vi "led_player.vi"() -> ()   [LabVIEW 2022 SP3]
uses:
  <vilib>/DAQmx/write.llb/DAQmx Write (Digital 1D Bool 1Chan 1Samp).vi
  <vilib>/DAQmx/create/channels.llb/DAQmx Create Channel (DO-Digital Output).vi
  <vilib>/DAQmx/create/channels.llb/DAQmx Create Channel (CO-Pulse Generation-Time).vi
  <vilib>/DAQmx/configure/trigger.llb/DAQmx Start Trigger (Digital Edge).vi
  <vilib>/DAQmx/miscellaneous.llb/DAQmx Fill In Error Info.vi
panel:
  in  "Numeric":i32
  out "Array":bool[](array[boolean])
  out "task done?":bool
  in  "counter":tag="cDAQ2/_ctr0"
  in  "source":tag="/cDAQ2/PFI0"
  in  "lines":tag="cDAQ2Mod3/port0/line0:3"
  in  "stop":bool
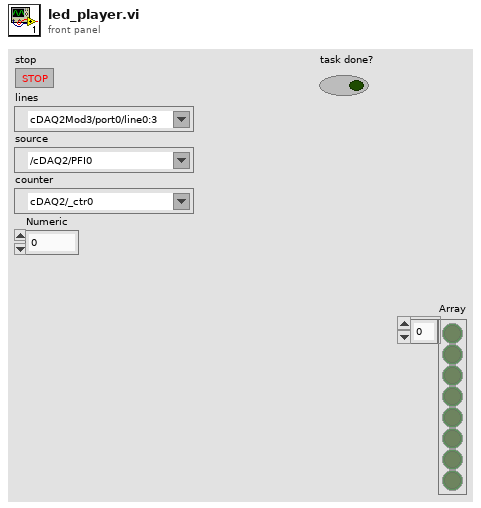
[diagram p1: front panel]
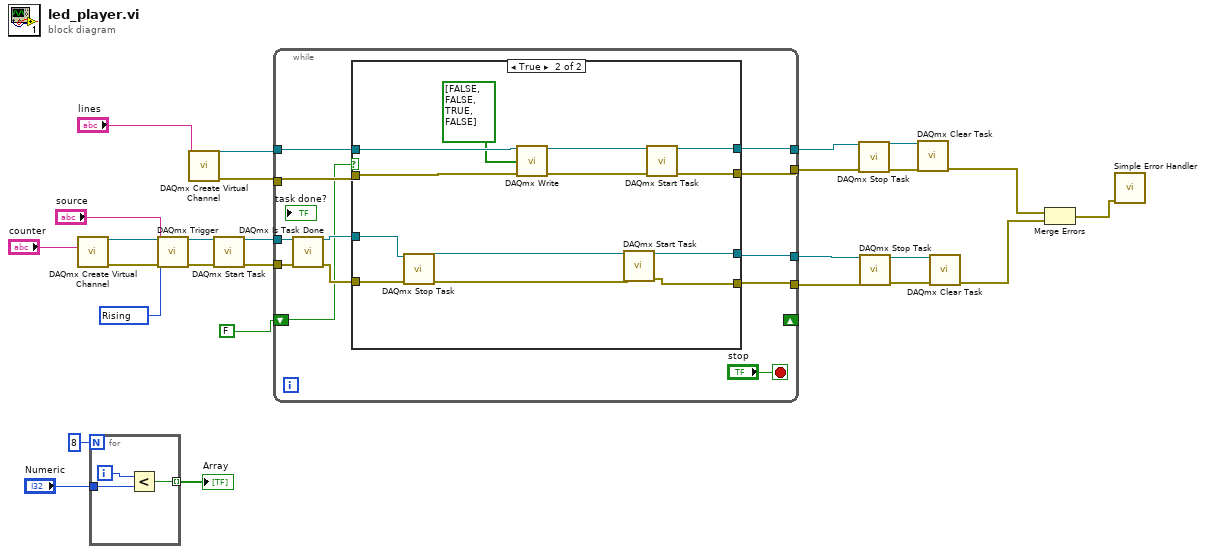
[diagram p0: block diagram]
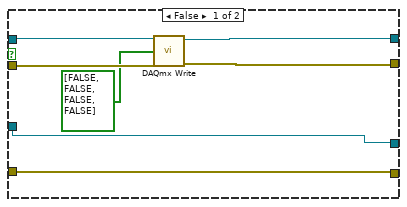
[diagram p2: hidden frame]
diagram:
  w6 = 10280 items=["Rising"=10280, "Falling"=10171] ("edge")
  n1 = call-poly <vilib>:"DAQmx Create Virtual Channel.vi"("counter"="counter") -> ("task out"=w16:refnum<k21>, "error out"=w27:errorcluster)  [unwired: 13 in]
  n2 = for {
    N: 8 -> [_]
    tunnel: "Numeric" -> [w29]
    tunnel: [w28] -> w3 mode=indexing
    i -> [w30]
    n3 = Less?(x=w30, y=w29) -> (x < y?=w28:bool)
  }
  "Array" <- w3
  n4 = call-poly <vilib>:"DAQmx Trigger.vi"("task/channels in"=w16, "source"="source", "edge"=w6, "error in"=w27) -> ("task out"=w17:refnum<k21>, "error out"=w26:errorcluster)  [unwired: 10 in]
  n5 = call-poly <vilib>:"DAQmx Create Virtual Channel.vi"("lines"="lines") -> ("task out"=w9:refnum<k21>, "error out"=w15:errorcluster)  [unwired: 13 in]
  n6 = call <vilib>:"DAQmx Start Task.vi"("task/channels in"=w17, "error in"=w26) -> ("task out"=w18:refnum<k21>, "error out"=w25:errorcluster)  [unwired: 12 in]
  n7 = while {
    tunnel: w25 -> [w42]
    tunnel: [w40] -> w24
    tunnel: [w39] -> w19
    tunnel: w18 -> [w37]
    tunnel: w15 -> [w36]
    tunnel: [w35] -> w14
    tunnel: [w34] -> w10
    tunnel: w9 -> [w33]
    shift-right: _ -> [_]
    shift-left: FALSE -> [w31]
    stop <- "stop" stop-if-true
    n8 = call <vilib>:"DAQmx Is Task Done.vi"("task/channels in"=w37, "error in"=w42) -> ("task out"=w38:refnum<k21>, "error out"=w41:errorcluster)  [unwired: 11 in, 1 out]
    n9 = case shown="True" w31 {
      tunnel: w41 -> [w47 w62]
      tunnel: [w47 w60] -> w40
      tunnel: [w46 w59] -> w39
      tunnel: w38 -> [w46 w57]
      tunnel: w36 -> [w48 w56]
      tunnel: [w44 w50] -> w35
      tunnel: [w45 w52] -> w34
      tunnel: w33 -> [w49 w55]
      frame False {
        n10 = call-poly <vilib>:"DAQmx Write.vi"("task/channels in"=w49, "data"=bool[] [FALSE, FALSE, FALSE, FALSE], "error in"=w48) -> ("task out"=w45:refnum<k21>, "error out"=w44:errorcluster)  [unwired: 10 in, 1 out]
      }
      frame True {
        n11 = call <vilib>:"DAQmx Stop Task.vi"("task/channels in"=w57, "error in"=w62) -> ("task out"=w58:refnum<k21>, "error out"=w61:errorcluster)  [unwired: 12 in]
        n12 = call-poly <vilib>:"DAQmx Write.vi"("task/channels in"=w55, "data"=bool[] [FALSE, FALSE, TRUE, FALSE], "error in"=w56) -> ("task out"=w53:refnum<k21>, "error out"=w51:errorcluster)  [unwired: 10 in, 1 out]
        n13 = call <vilib>:"DAQmx Start Task.vi"("task/channels in"=w58, "error in"=w61) -> ("task out"=w59:refnum<k21>, "error out"=w60:errorcluster)  [unwired: 12 in]
        n14 = call <vilib>:"DAQmx Start Task.vi"("task/channels in"=w53, "error in"=w51) -> ("task out"=w52:refnum<k21>, "error out"=w50:errorcluster)  [unwired: 12 in]
      }
    }
  }
  n15 = call <vilib>:"DAQmx Stop Task.vi"("task/channels in"=w10, "error in"=w14) -> ("task out"=w11:refnum<k21>, "error out"=w13:errorcluster)  [unwired: 12 in]
  n16 = call <vilib>:"DAQmx Stop Task.vi"("task/channels in"=w19, "error in"=w24) -> ("task out"=w20:refnum<k21>, "error out"=w23:errorcluster)  [unwired: 12 in]
  n17 = call <vilib>:"DAQmx Clear Task.vi"("task in"=w11, "error in"=w13) -> ("error out"=w12:errorcluster)  [unwired: 13 in]
  n18 = call <vilib>:"DAQmx Clear Task.vi"("task in"=w20, "error in"=w23) -> ("error out"=w22:errorcluster)  [unwired: 13 in]
  n19 = Merge Errors(w12, w22) -> (w21:errorcluster)
  n20 = call <vilib>:"Simple Error Handler.vi"("error in (no error)"=w21) -> ()  [unwired: 4 in, 5 out]
